vi "ROS_Master_WebPageServer.vi"(5 "occurrence":refnum<k4>) -> ()   [LabVIEW 2014]
doc: "Starts a server for the webpages"
uses:
  <userlib>/ROS for LabVIEW Software/ROS/Code/_ROSDefinition.vi
panel:
  out "requests":string[](array[string])
  out "Last Reply":string="HTTP/1.1 200 OK\r\nUser-Agent: LabVIEW WebServer/0.1\nDate: Thu, 08 Dec 2011 18:58:48 GMT\nExpires: Thu, 08 Dec 2011 18:58:48 GMT\nIgnore-Buffer: xXxBUFFERxXx\nContent-Type: text/html\nContent-Length: 508\nConnection: keep-alive\r\n\r\n<!DOCTYPE HTML PUBLIC \"-//W3C//DTD HTML 4.0 Transitional//EN\">\n<HTML>\n<!-- Constructed with LabVIEW Report Generation -->\n<HEAD>\n<TITLE></TITLE>\n</HEAD>\n\n<BODY>\n\n<form name=\"myform\" action=\"index.htm\" method=\"POST\">\n\n<br><br>\n____<input type=\"submit\" name=\"1\" value=\"forward\"> \n<br><br>\n<input type=\"submit\" name=\"2\" value=\"left\"> \n<input type=\"submit\" name=\"0\" value=\"STOP\"> \n<input type=\"submit\" name=\"3\" value=\"right\">\n<br><br>\n_____<input type=\"submit\" name=\"4\" value=\"back\"> \n\n</form>\n\n</BODY>\n\n</HTML>\r\n\r\n"
  in  "stop":bool
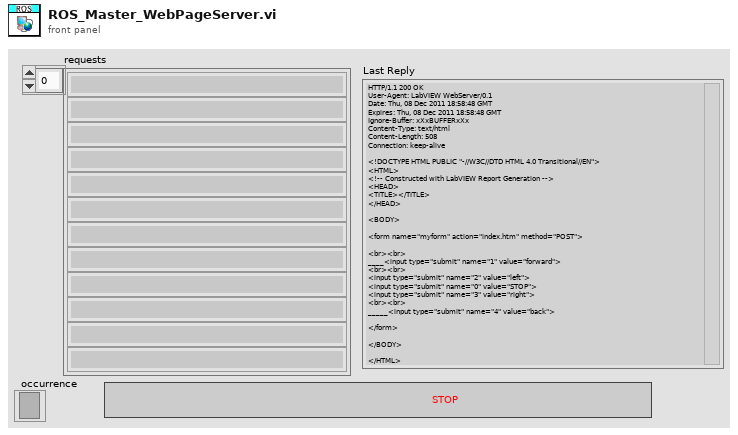
[diagram p1: front panel]
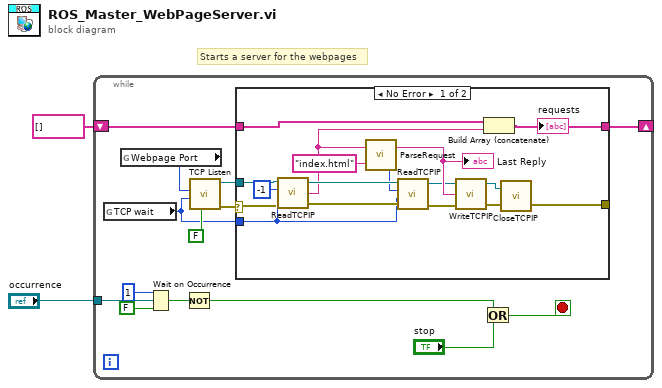
[diagram p0: block diagram]
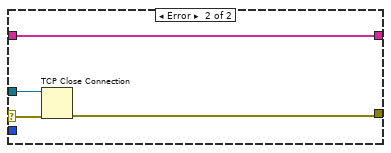
[diagram p2: hidden frame]
diagram:
  # "Starts a server for the webpages"
  n1 = while {
    shift-right: [w12] -> _
    shift-left: string[] [] -> [w11]
    tunnel: "occurrence" -> [w10]
    stop <- w5 stop-if-true
    n2 = global read "_ROSDefinition.vi" "TCP wait"() -> (w14:i32)
    n3 = global read "_ROSDefinition.vi" "Webpage Port"() -> (w13:u16)
    n4 = Wait on Occurrence(1:FALSE ("ignore previous (T)"), 2:w10, 3:1 ("ms timeout (-1)")) -> (0:w7:bool)
    n5 = Not(x=w7) -> (.not. x?=w4:bool)
    n6 = call <vilib>:"TCP Listen.vi"("resolve remote address (T)"=FALSE, "timeout ms (wait forever: -1)"=w14, "port"=w13) -> ("error out"=w3:errorcluster, "connection ID"=w15:refnum<k5>)  [unwired: 4 in, 3 out]
    n7 = case shown="No Error" w3 {
      selector: w3 -> [w17 w34]
      tunnel: w15 -> [w33 w36]
      tunnel: [w24 w35] -> _
      tunnel: w14 -> [w22 _]
      tunnel: [w19 w37] -> w12
      tunnel: w11 -> [w18 w37]
      frame No Error {
        n8 = call <userlib>:"ReadTCPIP.vi"("error in"=w17, "TCP Timeout"=w22, "bytes to read"=-1, "connection ID"=w33) -> ("errorout"=w27:errorcluster, "String"=w20:string, "connection ID Out"=w29:refnum<k5>)
        n9 = call <userlib>:"ParseRequest.vi"("Node html"="index.html", "String in"=w20) -> ("Post size"=w28:i32, "Reply"=w30:string)
        "Last Reply" <- w30
        n10 = call <userlib>:"ReadTCPIP.vi"("error in"=w27, "TCP Timeout"=w22, "bytes to read"=w28, "connection ID"=w29) -> ("errorout"=w26:errorcluster, "connection ID Out"=w25:refnum<k5>)  [unwired: 1 out]
        n11 = call <userlib>:"WriteTCPIP.vi"("error in"=w26, "String"=w30, "connection ID"=w25) -> ("errorout"=w32:errorcluster, "connection ID Out"=w31:refnum<k5>)  [unwired: 1 in]
        n12 = Build Array (concatenate)(w18, w20) -> (w19:string[])
        "requests" <- w19
        n13 = call <userlib>:"CloseTCPIP.vi"("error in (no error)"=w32, "connection ID"=w31) -> ("error out"=w24:errorcluster)  [unwired: 1 in]
      }
      frame Error {
        n14 = TCP Close Connection(connection ID=w36, error in (no error)=w34) -> (error out=w35:errorcluster)  [unwired: 1 in, 1 out]
      }
    }
    n15 = Or(x=w4, y="stop") -> (x .or. y?=w5:bool)
  }
